vi "SetHandlerDataStructure.vi"(8 "error in (no error)":errorcluster, 11 "DataHandler in":refnum<class "DataHandlerMYiTOPS.lvclass">) -> (0 "error out":errorcluster, 3 "DataHandler out":refnum<class "DataHandlerMYiTOPS.lvclass">)   [LabVIEW 2017, in "DataHandlerMYiTOPS.lvclass"]
uses:
  DataHandlerMYiTOPS.lvclass
  DataHandlerMYiTOPS.lvclass/DataHandlerMYiTOPS.ctl
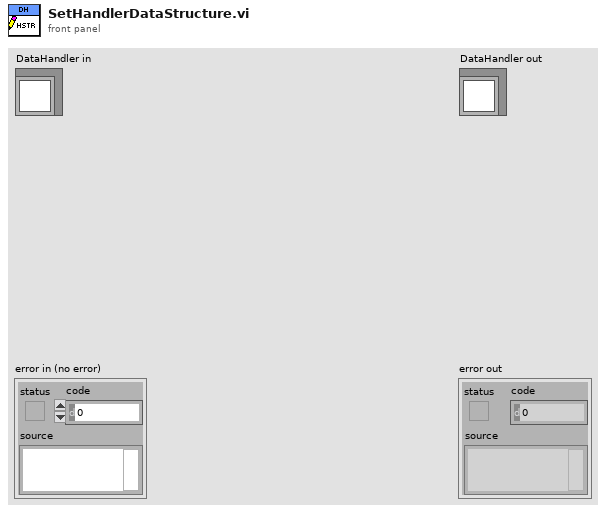
[diagram p1: front panel]
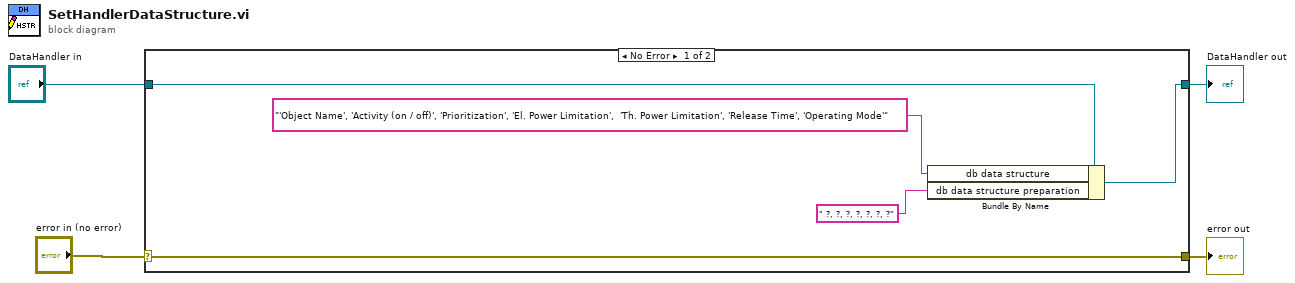
[diagram p0: block diagram]
diagram:
  n1 = case shown="No Error" "error in (no error)" {
    selector: "error in (no error)" -> [w9 w10]
    tunnel: [w9 w10] -> w3
    tunnel: [w7 w11] -> w1
    tunnel: "DataHandler in" -> [w8 w11]
    frame No Error {
      n2 = Bundle By Name(cluster=w8, "db data structure"="'Object Name', 'Activity (on / off)', 'Prioritization', 'El. Power Limitation',  'Th. Power Limitation', 'Release Time', 'Operating Mode'" ("string"), "db data structure preparation"=" ?, ?, ?, ?, ?, ?, ?") -> (w7:refnum<class "DataHandlerMYiTOPS.lvclass">)
    }
    frame Error {
    }
  }
  "error out" <- w3
  "DataHandler out" <- w1
